vi "Launch Dev List UI.vi"(8 "error in (no error)":errorcluster, 11 "Controller UI in":refnum<class "Controller UI.lvclass">) -> (0 "error out":errorcluster, 3 "Controller UI out":refnum<class "Controller UI.lvclass">)   [LabVIEW 2016, in "Controller UI.lvlib" / "Controller UI.lvclass"]
uses:
  <userlib>/Common Components/Controller UI/Controller UI.lvclass
  C:/Program Files (x86)/National Instruments/LabVIEW 2016/user.lib/Common Components/User Interface/UI.lvclass
  <userlib>/Common Components/Controller UI/Update DT event data.ctl
  <userlib>/Common Components/Controller UI/Update DT Cmd.ctl
  <userlib>/Common Components/Controller UI/Controller UI.lvclass/Controller UI.ctl
  <userlib>/Common Components/Controller UI/Accessors/Write Subpanel VI Refnum.vi
  <userlib>/Common Components/Controller UI/Accessors/Read Subpanel VI Refnum.vi
  <userlib>/Common Components/Controller UI/Accessors/Read HW_DEV Subpanel.vi
  <userlib>/Common Components/Controller UI/Accessors/Write Update DT event.vi
  <userlib>/Common Components/User Interface/UI.lvclass
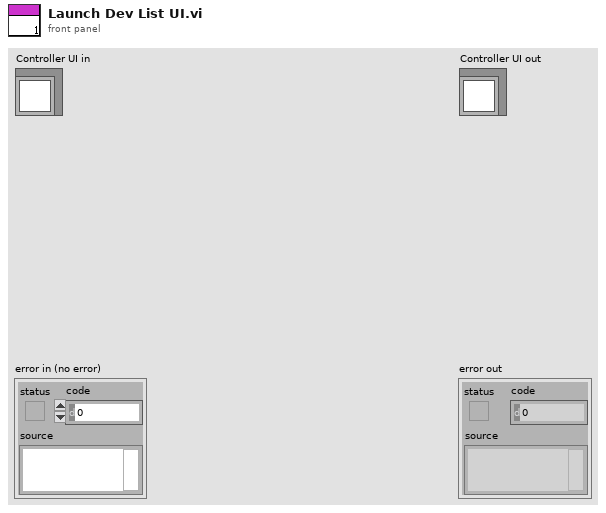
[diagram p1: front panel]
types:
  T1 = typedef "Controller UI.lvlib/Controller UI.lvclass/Update DT event data.ctl" = cluster{"Cmd":T2, "Data Array":variant[]}
  T2 = typedef "Controller UI.lvlib/Controller UI.lvclass/Update DT Cmd.ctl" = enum16{"Update HWtype\\HWplugin array", "Update Checked-out", "Update COMM Status", "Load DevInfo from File", "Save DevInfo to File", "Update COMM Address List"}
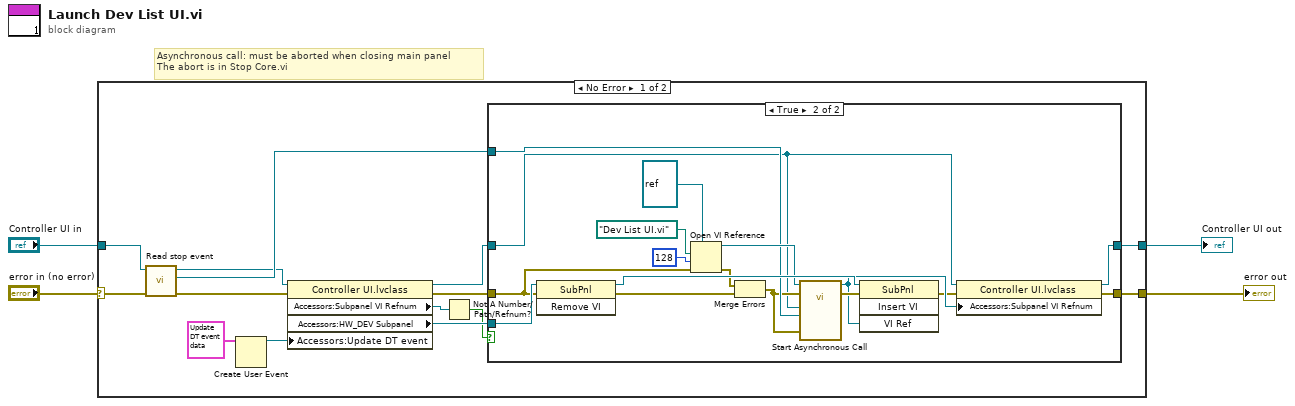
[diagram p0: block diagram]
diagram:
  # "Asynchronous call: must be aborted when closing main panel\nThe abort is in Stop Core.vi"
  n1 = case shown="No Error" "error in (no error)" {
    selector: "error in (no error)" -> [w15 w39]
    tunnel: [w10 w39] -> w3
    tunnel: [w17 w38] -> w1
    tunnel: "Controller UI in" -> [w18 w38]
    frame No Error {
      n2 = call <userlib>:"Read stop event.vi"("error in (no error)"=w15, "UI in"=w18) -> ("error out"=w11:errorcluster, "stop event"=w16:refnum<user-event>, "UI out"=w7:refnum<class "Controller UI.lvclass">)  [unwired: 7 in]
      n3 = Create User Event(user event datatype=T1 {"Cmd"=enum."Update HWtype\\HWplugin array", "Data Array"=[]} ("Update DT")) -> (user event=w5:refnum<user-event>)  [unwired: 1 in, 1 out]
      n4 = property class="Controller UI.lvclass"(reference=w7, error in=w11, "Accessors:Update DT event"=w5) -> (reference out=w14:refnum<class "Controller UI.lvclass">, error out=w12:errorcluster, "Accessors:Subpanel VI Refnum"=w9:refnum<vi>, "Accessors:HW_DEV Subpanel"=w13:refnum<vi>)
      n5 = Not A Number/Path/Refnum?(number/path/refnum=w9) -> (NaN/Path/Refnum?=w8:bool)
      n6 = case shown="True" w8 {
        tunnel: [w20 w29] -> w17
        tunnel: w16 -> [_ w28]
        tunnel: w14 -> [w20 w21]
        tunnel: w13 -> [_ w27]
        tunnel: w12 -> [w19 w22]
        tunnel: [w19 w23] -> w10
        frame False {
        }
        frame True {
          n7 = invoke class="SubPnl" method="Remove VI"(reference=w27, error in=w22) -> (reference out=w37:refnum<vi>, error out=w31:errorcluster)  [unwired: 1 in, 1 out]
          n8 = Open VI Reference(type specifier VI Refnum (for type only)=refnum<vi> refnum, vi path=path "Dev List UI.vi", options=128, error in (no error)=w22) -> (vi reference=w32:refnum<vi>, error out=w25:errorcluster)  [unwired: 2 in]
          n9 = Merge Errors(w25, w31) -> (w26:errorcluster)
          n10 = call-by-ref "Start Asynchronous Call"(reference=w32, error in=w26, 8:"error in (no error)"=w26, "stop event"=w28, "Operator UI in"=w21) -> (reference out=w30:refnum<vi>, error out=w36:errorcluster)  [unwired: 8 in, 1 out]
          n11 = invoke on="Invoke Node" class="SubPnl" method="Insert VI"(reference=w37, error in=w36, "VI Ref"=w30) -> (error out=w24:errorcluster)  [unwired: 1 in, 3 out]
          n12 = property class="Controller UI.lvclass"(reference=w21, error in=w24, "Accessors:Subpanel VI Refnum"=w30) -> (reference out=w29:refnum<class "Controller UI.lvclass">, error out=w23:errorcluster)
        }
      }
    }
    frame Error {
    }
  }
  "error out" <- w3
  "Controller UI out" <- w1
